vi "dual_chirp_wphase.vi"() -> ()   [LabVIEW 2014]
uses:
  <vilib>/Utility/file.llb/Read From Spreadsheet File (DBL).vi
  <vilib>/gmath/NI_Gmath.lvlib
panel:
  out "burleigh shift expected":dbl format="%#_13g"
  out "trek shift expected":dbl format="%#_13g"
  out "burleigh shift meas":dbl format="%#_13g"
  out "trek shift meas":dbl format="%#_13g"
  in  "Hz/step":dbl=-1.0
  in  "Stop Freq (Hz)":dbl=6000.0
  in  "Start Freq (Hz)":dbl=8000.0
  out "Current Freq":dbl format="%#_13g"
  in  "Step Length (s)":i32=5
  in  "Amplitude (V)":dbl=100.0
  in  "Manual Offset (V)":dbl=50.0
  in  "Auto Offset":bool=TRUE
  in  "Offset Trim (part per thousand)":i32
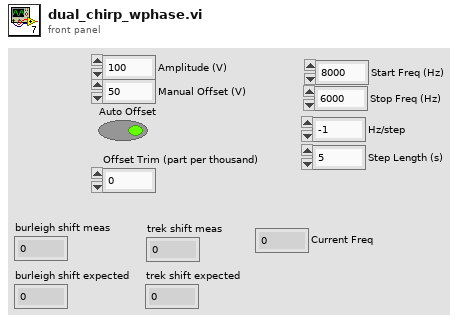
[diagram p1: front panel]
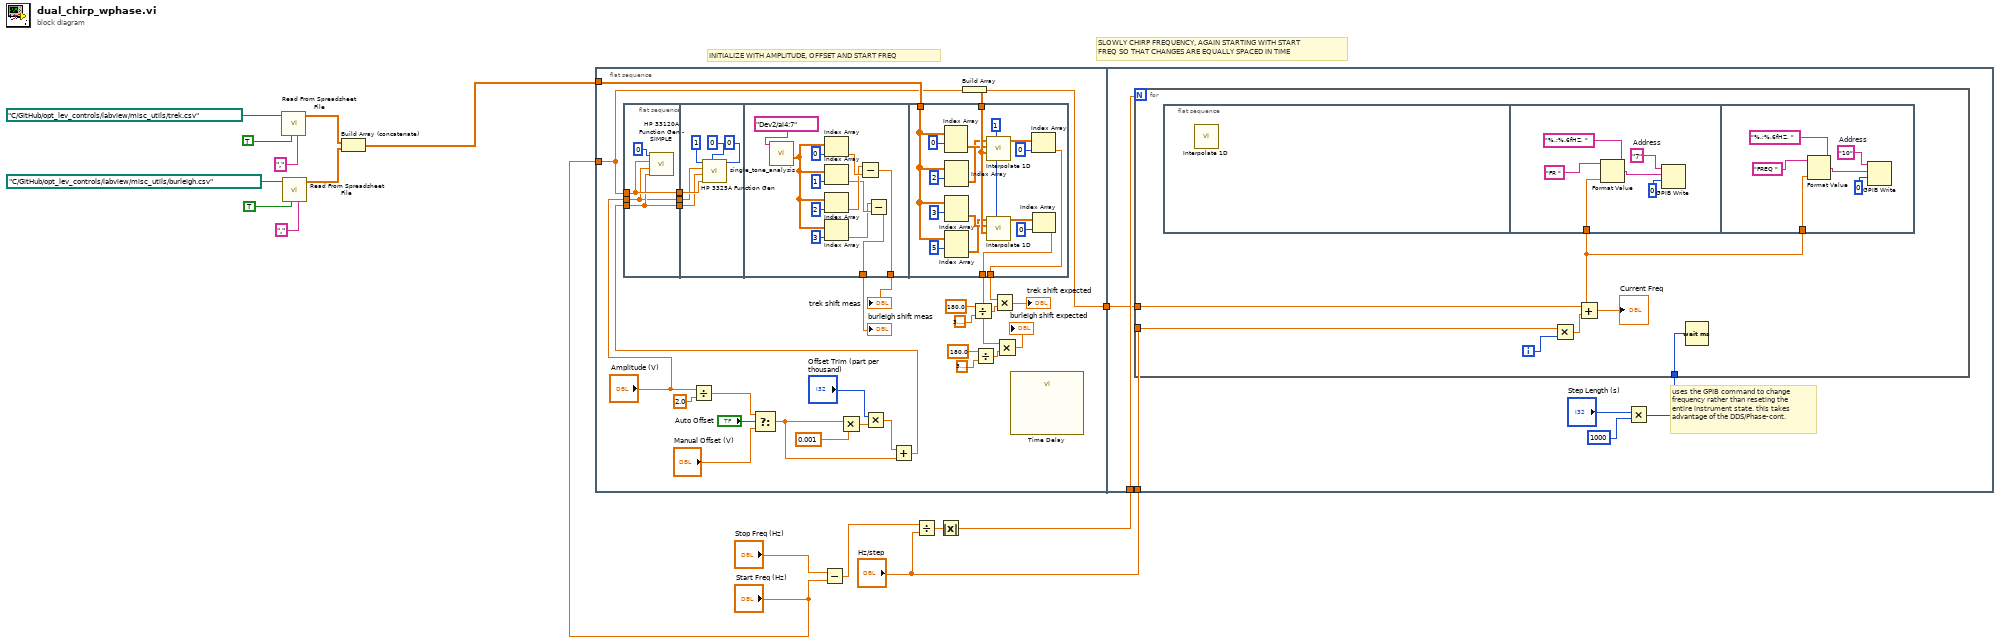
[diagram p0: block diagram]
diagram:
  # "SLOWLY CHIRP FREQUENCY, AGAIN STARTING WITH START\nFREQ SO THAT CHANGES ARE EQUALLY SPACED IN TIME"
  # "INITIALIZE WITH AMPLITUDE, OFFSET AND START FREQ"
  n1 = call-poly <vilib>:"Read From Spreadsheet File.vi"("delimiter (\\t)"=",", "transpose (no:F)"=TRUE, "file path (dialog if empty)"=path "C:/GitHub/opt_lev_controls/labview/misc_utils/trek.csv") -> ("all rows"=w3:dbl[][])  [unwired: 4 in, 4 out]
  n2 = call-poly <vilib>:"Read From Spreadsheet File.vi"("delimiter (\\t)"=",", "transpose (no:F)"=TRUE, "file path (dialog if empty)"=path "C:/GitHub/opt_lev_controls/labview/misc_utils/burleigh.csv") -> ("all rows"=w2:dbl[][])  [unwired: 4 in, 4 out]
  n3 = Build Array (concatenate)(w3, w2) -> (w1:dbl[][])
  n4 = flat-sequence {
    tunnel: "Start Freq (Hz)" -> [w30]
    tunnel: [w30] -> w16
    tunnel: w1 -> [w32]
    tunnel: w11 -> [w87]
    tunnel: "Hz/step" -> [w86]
    tunnel: w16 -> [w85]
    frame #0 {
      n5 = flat-sequence {
        tunnel: "Amplitude (V)" -> [w46]
        tunnel: w36 -> [w47]
        tunnel: w30 -> [w48]
        tunnel: [w48] -> w35
        tunnel: [w47] -> w34
        tunnel: [w46] -> w33
        tunnel: w35 -> [w52]
        tunnel: w34 -> [w51]
        tunnel: w33 -> [w50]
        tunnel: [w57] -> w28
        tunnel: [w56] -> w27
        tunnel: w32 -> [w76]
        tunnel: w31 -> [w83]
        tunnel: [w69] -> w18
        tunnel: [w68] -> w23
        frame #0 {
          n6 = call "HP 33120A Function Gen - SIMPLE.vi"("offset (V)"=w47, "amplitude (V)"=w46, "frequency (Hz)"=w48, "Function Type"=0) -> ()  [unwired: 8 in]
        }
        frame #1 {
          n7 = call "HP 3325A Function Gen.vi"("sweep function (none:0)"=0, "modulation (off:0)"=0, "frequency (Hz)"=w52, "offset (V)"=w51, "amplitude (V)"=w50, "signal type (dc:0)"=1) -> ()  [unwired: 4 in]
        }
        frame #2 {
          n8 = call "single_tone_analysis.vi"("channels"=tag "Dev2/ai4:7" ("Physical Channels (Position signals)")) -> ("Phases"=w67:dbl[])  [unwired: 8 in, 2 out]
          n9 = Index Array(array=w67, index=0) -> (element=w61:dbl)
          n10 = Index Array(array=w67, index=1) -> (element=w59:dbl)
          n11 = Index Array(array=w67, index=2) -> (element=w60:dbl)
          n12 = Index Array(array=w67, index=3) -> (element=w58:dbl)
          n13 = Subtract(x=w60, y=w61) -> (x-y=w57:dbl)
          n14 = Subtract(x=w58, y=w59) -> (x-y=w56:dbl)
        }
        frame #3 {
          w84 = 1
          n15 = Index Array(array=w76, index (row)=0) -> (element=w81:dbl[])  [unwired: 1 in]
          n16 = Index Array(array=w76, index (row)=2) -> (element=w77:dbl[])  [unwired: 1 in]
          n17 = Index Array(array=w76, index (row)=3) -> (element=w75:dbl[])  [unwired: 1 in]
          n18 = Index Array(array=w76, index (row)=5) -> (element=w74:dbl[])  [unwired: 1 in]
          n19 = call <vilib>:"Interpolate 1D.vi"("method"=w84, "xi"=w83, "X"=w81, "Y"=w77) -> ("yi"=w72:dbl[])  [unwired: 5 in, 2 out]
          n20 = call <vilib>:"Interpolate 1D.vi"("method"=w84, "xi"=w83, "X"=w75, "Y"=w74) -> ("yi"=w70:dbl[])  [unwired: 5 in, 2 out]
          n21 = Index Array(array=w72, index=0) -> (element=w69:dbl)
          n22 = Index Array(array=w70, index=0) -> (element=w68:dbl)
        }
      }
      n23 = Divide(x="Amplitude (V)", y=2.0) -> (x/y=w43:dbl)
      n24 = Select(t=w43, s="Auto Offset", f="Manual Offset (V)") -> (s? t:f=w41:dbl)
      n25 = Multiply(x=w41, y=0.001) -> (x*y=w38:dbl)
      n26 = Multiply(x="Offset Trim (part per thousand)", y=w38) -> (x*y=w37:dbl)
      n27 = Add(x=w37, y=w41) -> (x+y=w36:dbl)
      n28 = Build Array(w30) -> (w31:dbl[])
      n29 = Divide(x=180.0, y=3.141592653589793) -> (x/y=w19:dbl)
      n30 = Divide(x=180.0, y=3.141592653589793) -> (x/y=w26:dbl)
      n31 = Multiply(x=w18, y=w19) -> (x*y=→"trek shift expected":dbl)
      n32 = Multiply(x=w23, y=w26) -> (x*y=→"burleigh shift expected":dbl)
      n33 = call "Time Delay"() -> ()  [unwired: 11 in, 1 out]
      "trek shift meas" <- w28
      "burleigh shift meas" <- w27
    }
    frame #1 {
      # "uses the GPIB command to change\nfrequency rather than reseting the\nentire instrument state. this takes\nadvantage of the DDS/Phase-cont."
      n34 = Multiply(x="Step Length (s)", y=1000) -> (x*y=w90:i32)
      n35 = for {
        N: w87 -> [_]
        tunnel: w85 -> [w95]
        tunnel: w86 -> [w96]
        tunnel: w90 -> [w92]
        i -> [w93]
        n36 = flat-sequence {
          tunnel: w91 -> [w97]
          tunnel: w91 -> [w103]
          frame #0 {
            n37 = call <vilib>:"Interpolate 1D.vi"() -> ()  [unwired: 9 in, 3 out]
          }
          frame #1 {
            w101 = "7"  # Address
            n38 = Format Value(string ("")="FR ", format string="%.;%.6fHZ, ", value (0)=w97) -> (output string=w98:string)
            n39 = GPIB Write(0:w101, 1:w98, 2:0) -> ()  [unwired: 1 in, 3 out]
          }
          frame #2 {
            w105 = "10"  # Address
            n40 = Format Value(string ("")="FREQ ", format string="%.;%.6fHZ, ", value (0)=w103) -> (output string=w108:string)
            n41 = GPIB Write(0:w105, 1:w108, 2:0) -> ()  [unwired: 1 in, 3 out]
          }
        }
        n42 = Multiply(x=w96, y=w93) -> (x*y=w94:dbl)
        n43 = Add(x=w95, y=w94) -> (x+y=w91:dbl)
        "Current Freq" <- w91
        n44 = Wait (ms)(milliseconds to wait=w92) -> ()  [unwired: 1 out]
      }
    }
  }
  n45 = Subtract(x="Stop Freq (Hz)", y="Start Freq (Hz)") -> (x-y=w14:dbl)
  n46 = Divide(x=w14, y="Hz/step") -> (x/y=w13:dbl)
  n47 = Absolute Value(x=w13) -> (abs(x)=w11:dbl)
